vi "2Dscan_line-by-line.vi"(4 "stop":bool, 5 "IntGraph Refnum":refnum<vi>, 6 "XY Window Size (V)":dbl=0.015, 7 "scan mode":u16(ring) items=["unidirectional", "zig-zag"], 8 "Number of X/Y steps":i32=20, 9 "time per point (s)":dbl=0.02 format="%#_6p", 10 "Y Start (V)":dbl=-0.24561810526315794, 11 "X Start (V)":dbl=0.3860729041916167) -> (1 "Y scale":dbl[](array[numeric])=[-0.24561810526315794, -0.24486810526315794, -0.24411810526315794, -0.24336810526315794, -0.24261810526315794, -0.24186810526315794, -0.24111810526315794, -0.24036810526315794, -0.23961810526315794, -0.23886810526315794, -0.23811810526315796, -0.23736810526315796, -0.23661810526315796, -0.23586810526315796, -0.23511810526315796, -0.23436810526315796, -0.23361810526315796, -0.23286810526315796, -0.23211810526315796, -0.23136810526315796], 2 "X scale":dbl[](array[numeric])=[0.3860729041916167, 0.3868229041916167, 0.3875729041916167, 0.38832290419161675, 0.3890729041916167, 0.3898229041916167, 0.3905729041916167, 0.39132290419161675, 0.3920729041916167, 0.3928229041916167, 0.3935729041916167, 0.39432290419161675, 0.3950729041916167, 0.3958229041916167, 0.3965729041916167, 0.39732290419161675, 0.3980729041916167, 0.3988229041916167, 0.39957290419161673, 0.40032290419161676], 3 "Intensity Graph (counts/s)":dbl[][](graph)=[[56900.0, 73100.0, 60800.0, 70900.0, 93900.0, 93900.0, 101900.0, 121400.0, 114300.0, 94200.0, 101600.0, 84300.0, 76200.0, 51400.0, 56800.0, 76400.0, 52800.0, 48600.0, 60100.0, 63800.0], [49900.0, 56600.0, 68100.0, 73500.0, 67900.0, 82100.0, 85300.0, 88700.0, 95600.0, 90800.0, 101800.0, 79600.0, 58500.0, 87900.0, 53100.0, 48700.0, 82800.0, 54600.0, 67600.0, 51900.0], [51500.0, 53700.0, 66500.0, 70500.0, 77500.0, 127700.0, 74500.0, 78500.0, 83700.0, 78500.0, 68400.0, 77000.0, 64400.0, 58600.0, 49800.0, 53600.0, 54300.0, 84500.0, 55300.0, 69900.0], [53300.0, 67900.0, 59000.0, 55200.0, 56800.0, 59400.0, 63600.0, 74500.0, 76700.0, 69900.0, 74600.0, 71800.0, 56900.0, 66800.0, 57500.0, 60300.0, 64600.0, 54200.0, 52700.0, 68500.0], [52700.0, 59900.0, 61700.0, 52100.0, 69200.0, 82400.0, 58700.0, 78200.0, 79300.0, 79500.0, 80600.0, 80500.0, 74600.0, 63200.0, 76500.0, 50800.0, 47800.0, 46700.0, 50800.0, 59700.0], [64500.0, 63300.0, 50300.0, 43500.0, 49100.0, 54100.0, 61200.0, 67300.0, 86300.0, 81000.0, 93400.0, 84200.0, 76800.0, 70000.0, 92400.0, 51100.0, 48600.0, 57900.0, 73600.0, 56600.0], [52600.0, 51100.0, 42900.0, 65800.0, 53400.0, 58800.0, 71700.0, 86200.0, 112300.0, 133900.0, 147900.0, 139200.0, 116100.0, 106600.0, 73000.0, 60600.0, 81300.0, 55300.0, 56300.0, 87400.0], [47300.0, 46800.0, 51500.0, 60900.0, 59400.0, 81500.0, 75100.0, 95400.0, 105500.0, 113700.0, 127600.0, 126300.0, 122400.0, 114300.0, 120800.0, 72100.0, 68300.0, 45000.0, 51200.0, 43800.0], [48000.0, 85800.0, 97700.0, 48300.0, 62100.0, 63200.0, 78700.0, 106400.0, 133900.0, 134600.0, 133500.0, 134200.0, 131500.0, 113500.0, 80600.0, 71400.0, 59200.0, 55000.0, 53100.0, 54600.0], [57600.0, 48200.0, 68500.0, 45600.0, 67300.0, 77900.0, 102000.0, 103400.0, 128600.0, 143000.0, 134600.0, 140100.0, 128800.0, 114000.0, 106800.0, 108300.0, 72200.0, 61200.0, 81700.0, 53800.0], [46000.0, 46500.0, 49400.0, 66700.0, 80000.0, 79000.0, 89800.0, 105200.0, 121000.0, 150900.0, 142800.0, 157800.0, 122500.0, 117400.0, 94700.0, 70700.0, 64100.0, 59400.0, 70700.0, 52800.0], [46500.0, 45200.0, 53900.0, 46100.0, 50200.0, 65500.0, 85500.0, 103000.0, 118300.0, 131200.0, 138600.0, 138900.0, 140400.0, 105200.0, 88600.0, 65700.0, 60500.0, 67000.0, 67600.0, 55200.0], [64400.0, 83800.0, 67800.0, 54700.0, 97300.0, 61200.0, 77800.0, 95800.0, 118400.0, 117900.0, 156000.0, 130700.0, 116500.0, 94800.0, 108300.0, 70300.0, 59800.0, 51900.0, 51800.0, 53200.0], [73600.0, 61300.0, 65500.0, 54200.0, 57700.0, 59800.0, 72900.0, 102400.0, 153700.0, 146700.0, 109000.0, 107300.0, 99600.0, 104300.0, 103600.0, 84500.0, 59800.0, 45800.0, 52100.0, 48200.0], [48500.0, 51500.0, 52400.0, 76000.0, 64000.0, 71000.0, 86800.0, 92200.0, 93900.0, 93200.0, 96600.0, 93900.0, 78900.0, 66300.0, 58800.0, 68700.0, 46600.0, 43100.0, 54200.0, 54900.0], [58600.0, 59500.0, 53800.0, 59200.0, 57500.0, 63500.0, 66800.0, 73900.0, 83800.0, 78900.0, 80100.0, 79400.0, 75700.0, 64900.0, 115800.0, 43700.0, 64800.0, 47800.0, 52900.0, 60400.0], [54700.0, 50600.0, 51700.0, 63800.0, 82800.0, 74600.0, 74500.0, 84400.0, 81000.0, 78500.0, 91600.0, 77200.0, 87100.0, 57700.0, 54600.0, 54500.0, 45900.0, 44200.0, 51100.0, 50600.0], [56300.0, 60900.0, 51000.0, 59500.0, 68300.0, 71600.0, 68300.0, 84900.0, 76100.0, 75000.0, 84800.0, 77000.0, 64100.0, 54100.0, 52900.0, 52000.0, 63700.0, 53800.0, 47000.0, 54400.0], [46700.0, 82800.0, 61900.0, 54800.0, 64200.0, 67400.0, 71400.0, 70300.0, 91800.0, 124100.0, 80600.0, 89200.0, 59600.0, 58400.0, 59200.0, 54100.0, 48300.0, 53200.0, 51900.0, 60900.0], [79800.0, 84400.0, 86400.0, 84400.0, 67300.0, 70300.0, 83300.0, 79100.0, 73900.0, 82500.0, 75100.0, 79600.0, 72300.0, 70600.0, 65000.0, 80200.0, 46300.0, 66100.0, 104100.0, 48800.0]])   [LabVIEW 2014]
uses:
  <vilib>/Analysis/1siggen.llb/Ramp Pattern by Samples.vi
  global_channels.vi
  <vilib>/Analysis/NI_AALBase.lvlib
panel:
  out "discard graph":bool
  in  "stop and discard":bool
  out "time per line (s)":dbl=0.2 format="%#_6p"
  out "time left (s)":dbl
  out "Progress Bar":dbl(slide)=1.0 scale=0.0..1.0
  out "total time (s)":dbl=4.0
  out "X End (V)":dbl=0.40107290419161673
  out "Y End (V)":dbl=-0.23061810526315796
  out "X/Y Step Size (V)":dbl=0.00075
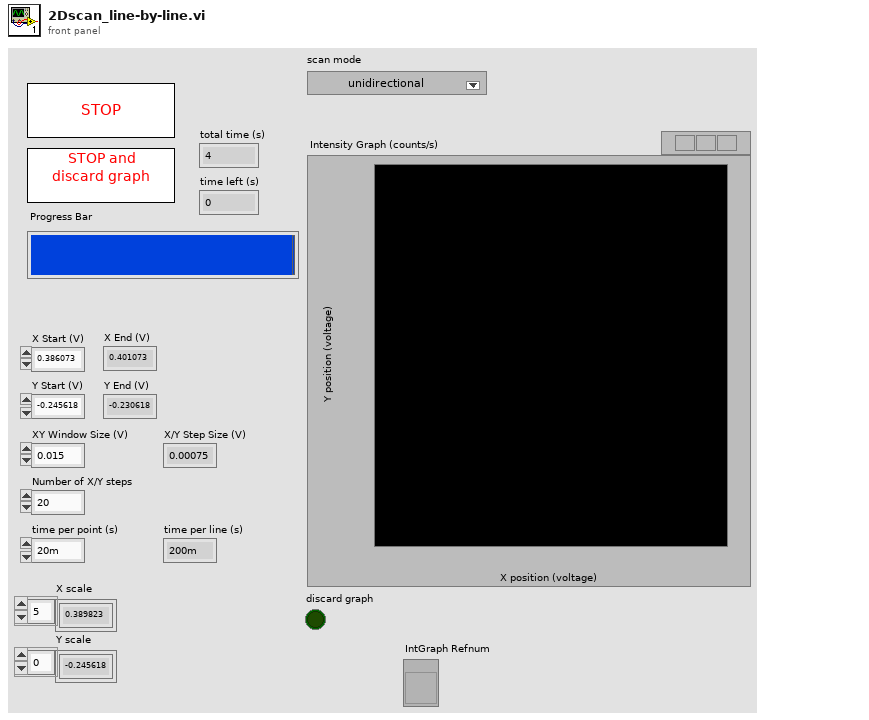
[diagram p1: front panel]
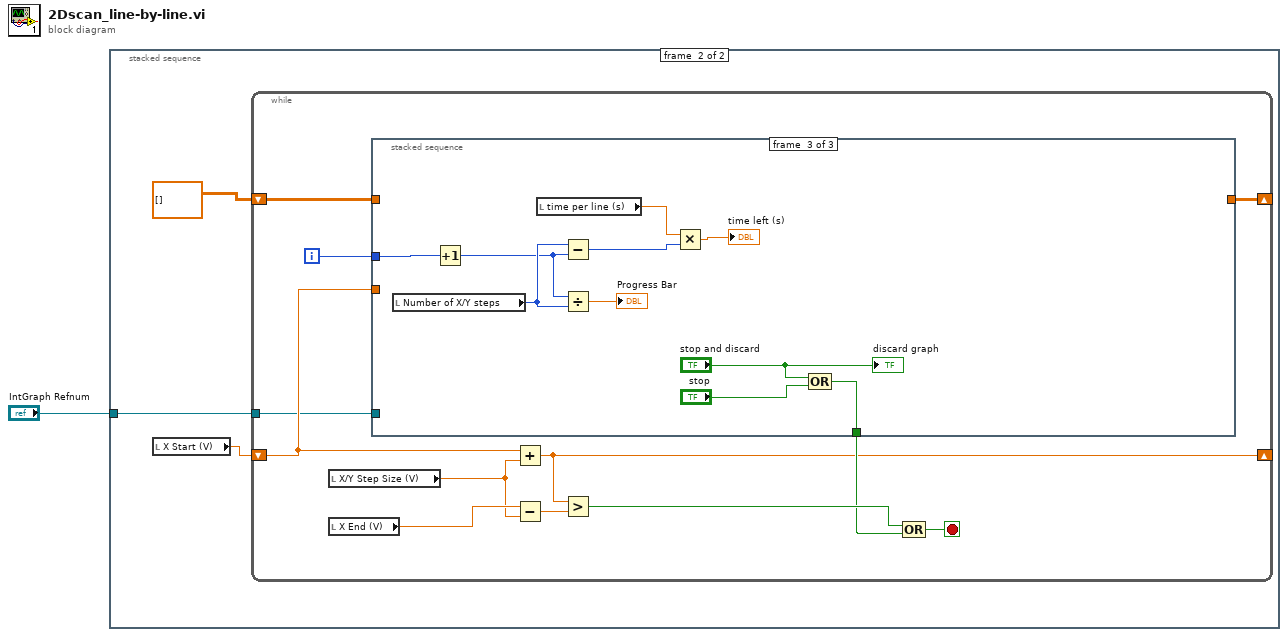
[diagram p0: block diagram]
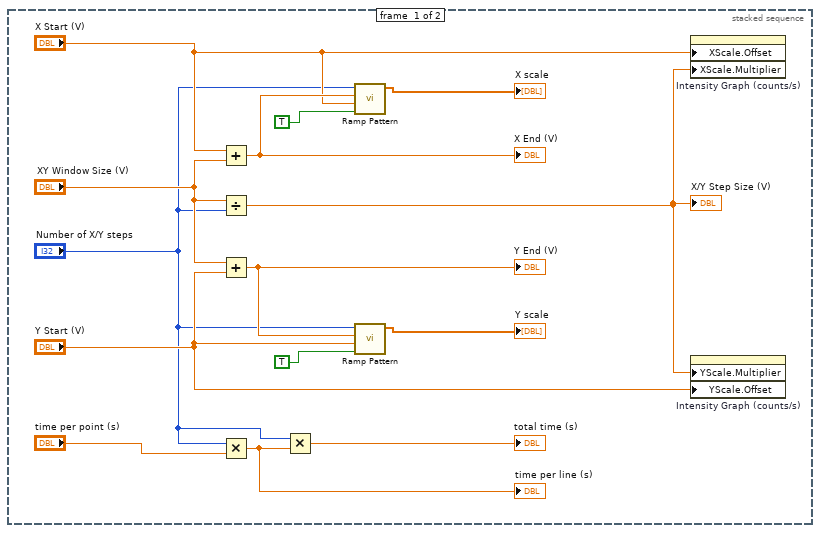
[diagram p2: hidden frame]
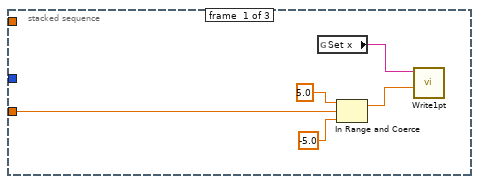
[diagram p3: hidden frame]
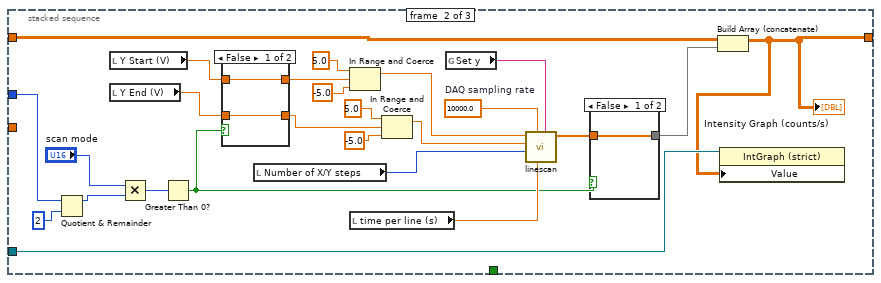
[diagram p4: hidden frame]
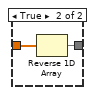
[diagram p5: hidden frame]
diagram:
  n1 = stacked-sequence {
    tunnel: "IntGraph Refnum" -> [_ w16]
    frame #0 {
      n2 = Add(x="X Start (V)", y="XY Window Size (V)") -> (x+y=w13:dbl)
      "X End (V)" <- w13
      n3 = Divide(x="XY Window Size (V)", y="Number of X/Y steps") -> (x/y=w15:dbl)
      "X/Y Step Size (V)" <- w15
      n4 = Add(x="XY Window Size (V)", y="Y Start (V)") -> (x+y=w10:dbl)
      "Y End (V)" <- w10
      n5 = Multiply(x="Number of X/Y steps", y="time per point (s)") -> (x*y=w6:dbl)
      "time per line (s)" <- w6
      n6 = Multiply(x="Number of X/Y steps", y=w6) -> (x*y=→"total time (s)":dbl)
      n7 = call-poly <vilib>:"Ramp Pattern.vi"("exclude end?"=TRUE, "start"="X Start (V)", "end"=w13, "samples"="Number of X/Y steps") -> ("Ramp Pattern"=→"X scale":dbl[])  [unwired: 6 in, 1 out]
      n8 = call-poly <vilib>:"Ramp Pattern.vi"("exclude end?"=TRUE, "start"="Y Start (V)", "end"=w10, "samples"="Number of X/Y steps") -> ("Ramp Pattern"=→"Y scale":dbl[])  [unwired: 6 in, 1 out]
      n9 = property on="Intensity Graph (counts/s)" class="IntGraph (strict)"("XScale.Offset"="X Start (V)", "XScale.Multiplier"=w15) -> ()  [unwired: 2 in, 2 out]
      n10 = property on="Intensity Graph (counts/s)" class="IntGraph (strict)"("YScale.Multiplier"=w15, "YScale.Offset"="Y Start (V)") -> ()  [unwired: 2 in, 2 out]
    }
    frame #1 {
      n11 = local read "X Start (V)"() -> (w18:dbl)
      n12 = while {
        shift-right: [w20] -> _
        shift-left: w18 -> [w21]
        shift-right: [w27] -> _
        shift-left: dbl[][] [] -> [w28]
        tunnel: w16 -> [w19]
        i -> [w23]
        stop <- w29 stop-if-true
        n13 = local read "X/Y Step Size (V)"() -> (w22:dbl)
        n14 = local read "X End (V)"() -> (w26:dbl)
        n15 = stacked-sequence {
          tunnel: w21 -> [w31 _ _]
          tunnel: w28 -> [_ w52 _]
          tunnel: [_ w36 _] -> w27
          tunnel: [_ _ w73] -> w24
          tunnel: w23 -> [_ w45 w77]
          tunnel: w19 -> [_ w37 _]
          frame #0 {
            n16 = global read "global_channels.vi" "Set x"() -> (w35:tag)
            n17 = In Range and Coerce(upper limit=5.0, x=w31, lower limit=-5.0) -> (coerced(x)=w34:dbl)  [unwired: 1 out]
            n18 = call "Write1pt.vi"("data"=w34, "physical channel"=w35) -> ()  [unwired: 10 in]
          }
          frame #1 {
            w53 = 10000.0  # DAQ sampling rate
            n19 = Quotient & Remainder(x=w45, y=2) -> (x-y*floor(x/y)=w40:i32)  [unwired: 1 out]
            n20 = local read "Y Start (V)"() -> (w46:dbl)
            n21 = local read "Y End (V)"() -> (w48:dbl)
            n22 = Multiply(x="scan mode", y=w40) -> (x*y=w39:i32)
            n23 = Greater Than 0?(x=w39) -> (x > 0?=w44:bool)
            n24 = case shown="False" w44 {
              tunnel: [w65 w67] -> w49
              tunnel: w48 -> [w65 w66]
              tunnel: [w64 w66] -> w47
              tunnel: w46 -> [w64 w67]
              frame False {
              }
              frame True {
              }
            }
            n25 = local read "Number of X/Y steps"() -> (w54:i32)
            n26 = In Range and Coerce(upper limit=5.0, x=w47, lower limit=-5.0) -> (coerced(x)=w56:dbl)  [unwired: 1 out]
            n27 = local read "time per line (s)"() -> (w50:dbl)
            n28 = In Range and Coerce(upper limit=5.0, x=w49, lower limit=-5.0) -> (coerced(x)=w55:dbl)  [unwired: 1 out]
            n29 = global read "global_channels.vi" "Set y"() -> (w51:tag)
            n30 = call "linescan.vi"("DAQ analog output"=w51, "duration"=w50, "DAQ sampling rate"=w53, "#counter bins"=w54, "analog output voltage2"=w55, "analog output voltage1"=w56) -> ("histogram plot"=w43:dbl[])  [unwired: 4 in, 1 out]
            n31 = case shown="False" w44 {
              tunnel: w43 -> [w61 w63]
              tunnel: [w61 w62] -> w42
              frame False {
              }
              frame True {
                n32 = Reverse 1D Array(array=w63) -> (reversed array=w62:dbl[])
              }
            }
            n33 = Build Array (concatenate)(w52, w42) -> (w36:dbl[][])
            "Intensity Graph (counts/s)" <- w36
            n34 = property class="IntGraph (strict)"(reference=w37, "Value"=w36) -> ()  [unwired: 1 in, 2 out]
          }
          frame #2 {
            n35 = local read "Number of X/Y steps"() -> (w75:i32)
            n36 = Increment(x=w77) -> (x+1=w74:i32)
            n37 = local read "time per line (s)"() -> (w70:dbl)
            n38 = Subtract(x=w75, y=w74) -> (x-y=w69:i32)
            n39 = Divide(x=w74, y=w75) -> (x/y=→"Progress Bar":dbl)
            n40 = Multiply(x=w70, y=w69) -> (x*y=→"time left (s)":dbl)
            n41 = Compound Arithmetic op=OR("stop and discard", "stop") -> (w73:bool)
            "discard graph" <- "stop and discard"
          }
        }
        n42 = Add(x=w21, y=w22) -> (x+y=w20:dbl)
        n43 = Subtract(x=w26, y=w22) -> (x-y=w25:dbl)
        n44 = Greater?(x=w20, y=w25) -> (0:w30:bool)
        n45 = Compound Arithmetic op=OR(w30, w24) -> (w29:bool)
      }
    }
  }
